vi "Crusher.vi"(8 "error in (no error)":errorcluster, 10 "Audio Data In":dbl[][](array[numeric]), 11 "Effect in":refnum<class "Effect.lvclass">) -> (0 "error out":errorcluster, 2 "Audio Data Out":dbl[][](array[numeric]), 3 "Effect out":refnum<class "Effect.lvclass">)   [LabVIEW 2018, in "Effect.lvclass"]
uses:
  Effect.lvclass
  Effect.lvclass/Effect.ctl
  <vilib>/Analysis/2dsp.llb/Decimate (single shot, DBL).vi
  <vilib>/gmath/NI_Gmath.lvlib
  <vilib>/Analysis/NI_AALPro.lvlib
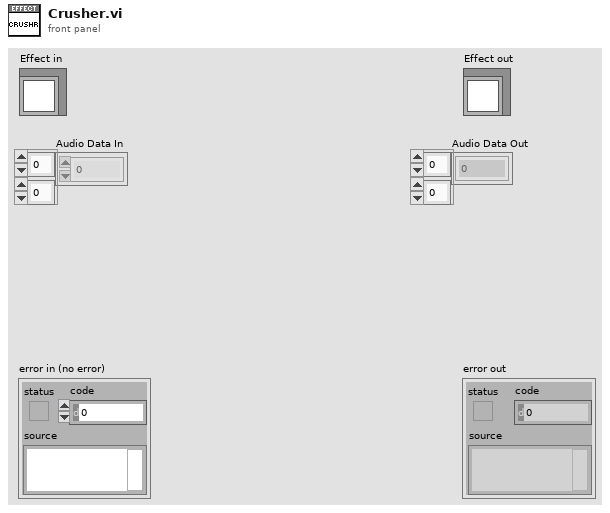
[diagram p1: front panel]
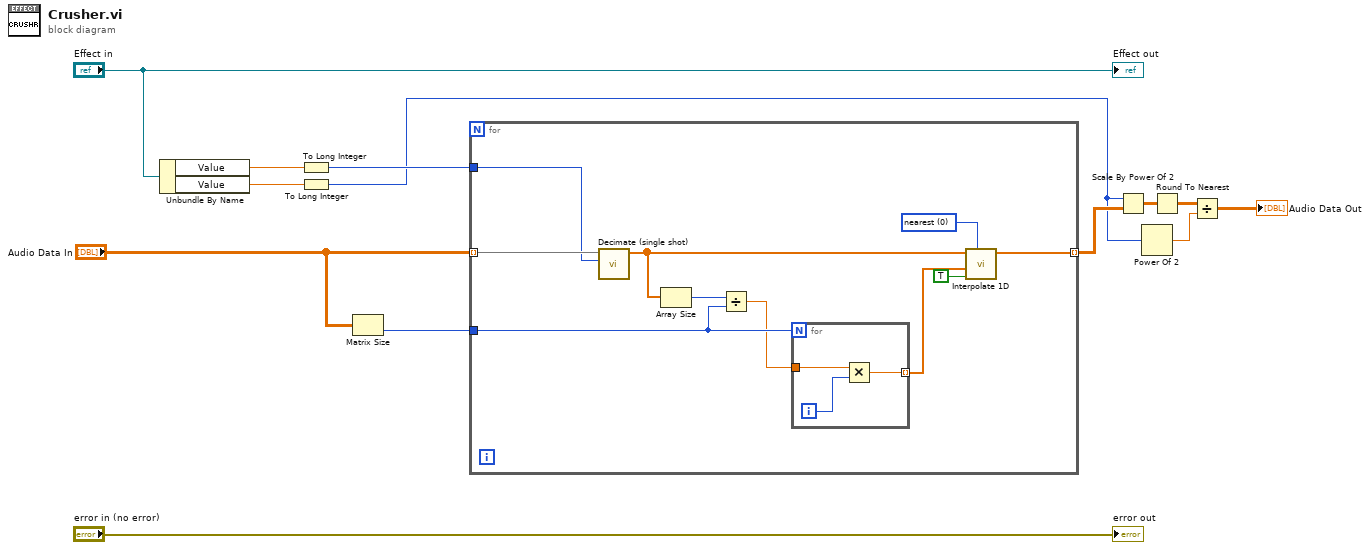
[diagram p0: block diagram]
diagram:
  n1 = Unbundle By Name("Effect in") -> ("Value"=w6:dbl, "Value"=w5:dbl)
  n2 = To Long Integer(number=w6) -> (32bit integer=w2:i32)
  n3 = To Long Integer(number=w5) -> (32bit integer=w1:i32)
  n4 = Matrix Size(0:"Audio Data In") -> (2:w12:i32)  [unwired: 1 out]
  n5 = for {
    tunnel: "Audio Data In" -> [w23] mode=indexing
    tunnel: w2 -> [w22]
    tunnel: w12 -> [w20]
    tunnel: [w14] -> w11 mode=indexing
    w15 = 0 items=["nearest", "linear", "spline", "cubic Hermite", "Lagrange"] ("method")
    n6 = call-poly <vilib>:"Decimate (single shot).vi"("decimating factor"=w22, "X"=w23) -> ("Decimated Array"=w16:dbl[])  [unwired: 8 in, 1 out]
    n7 = Array Size(array=w16) -> (size(s)=w21:i32)
    n8 = Divide(x=w21, y=w20) -> (x/y=w19:dbl)
    n9 = for {
      N: w20 -> [_]
      tunnel: w19 -> [w26]
      tunnel: [w24] -> w18 mode=indexing
      i -> [w25]
      n10 = Multiply(x=w26, y=w25) -> (x*y=w24:dbl)
    }
    n11 = call <vilib>:"Interpolate 1D.vi"("method"=w15, "X is monotonic"=TRUE, "xi"=w18, "Y"=w16) -> ("yi"=w14:dbl[])  [unwired: 5 in, 2 out]
  }
  n12 = Scale By Power Of 2(n=w1, x=w11) -> (x*2^n=w10:dbl[][])
  n13 = Power Of 2(x=w1) -> (2^x=w8:dbl)
  n14 = Round To Nearest(number=w10) -> (nearest integer value=w9:dbl[][])
  n15 = Divide(x=w9, y=w8) -> (x/y=→"Audio Data Out":dbl[][])
  "error out" <- "error in (no error)"
  "Effect out" <- "Effect in"
